vi "Flatten Value.vi"(8 "error in (no error)":errorcluster, 11 "Boolean in":refnum<class "String 1D.lvclass">) -> (0 "error out":errorcluster, 2 "Value":string, 3 "Boolean out":refnum<class "String 1D.lvclass">)   [LabVIEW 2020, in "String 1D.lvclass"]
uses:
  <vilib>/gpm_packages/@cs/data-type-serializer/source/String 1D/String 1D.lvclass
  <vilib>/gpm_packages/@cs/data-type-serializer/source/String 1D/String 1D.lvclass/String 1D.ctl
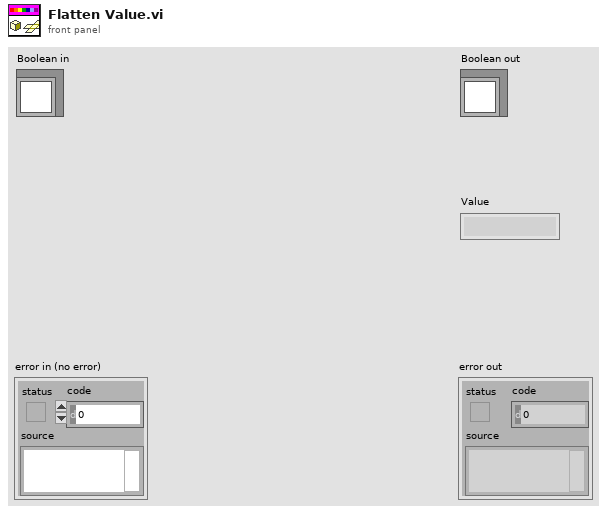
[diagram p1: front panel]
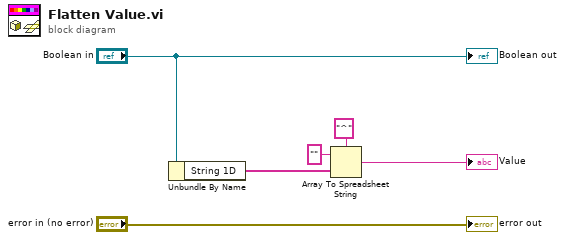
[diagram p0: block diagram]
diagram:
  n1 = Unbundle By Name("Boolean in") -> ("String 1D"=w3:string[])
  n2 = Array To Spreadsheet String(delimiter (Tab)="^", array=w3, 3:"" ("format string")) -> (spreadsheet string=→"Value":string)
  "error out" <- "error in (no error)"
  "Boolean out" <- "Boolean in"
